vi "Scale Potentiometer (subVI).vi"() -> (0 "Wait (us)":fxp<+/-,42,21> format="%.28g")   [LabVIEW 2015]
doc: "This VI samples the potentiometer on the sbRIO evaluation board and scales the value to an appropriate wait time. This will be used as a period control in the look-up table application."
uses:
  <vilib>/rvi/eio/common/nirviEmuTemplateMethod_errors.vi
  <vilib>/eio/EIONode/EIONode.xnode
panel:
  out "Pot Value":fxp<+/-,26,5> format="%.23g"
  # "This VI samples the potentiometer on the evaluation board and scales the value to an appropriate wait time.  This will be used as a period control in the look-up table application."
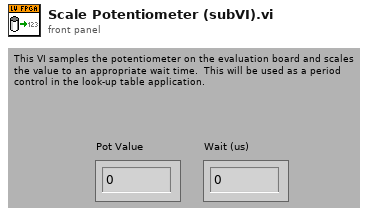
[diagram p1: front panel]
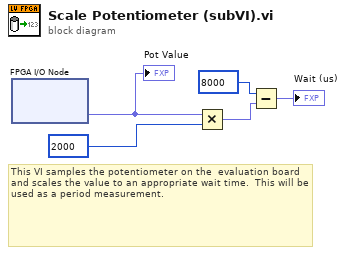
[diagram p0: block diagram]
diagram:
  # "This VI samples the potentiometer on the  evaluation board and scales the value to an appropriate wait time.  This will be used as a period measurement."
  n1 = xnode "FPGA I/O Node"() -> ("POT"=w3:fxp<+/-,24,5>)  [unwired: 1 in, 1 out]
  "Pot Value" <- w3
  n2 = Multiply(x=w3, y=i16 2000) -> (x*y=w5:fxp<+/-,40,21>)
  n3 = Subtract(x=i16 8000, y=w5) -> (x-y=→"Wait (us)":fxp<+/-,40,21>)
